vi "Append Goal.vi"(5 "Month":T1, 7 "YYYY":i32, 8 "error in (no error)":errorcluster, 9 "Goal Amount":dbl, 10 "Category_id":i32, 11 "Database in":refnum<class "Account History.lvclass">) -> (0 "error out":errorcluster, 2 "Added?":bool, 3 "Database out":refnum<class "Account History.lvclass">)   [LabVIEW 2018, in "Account History.lvclass"]
uses:
  Account History.lvclass
  Month.ctl
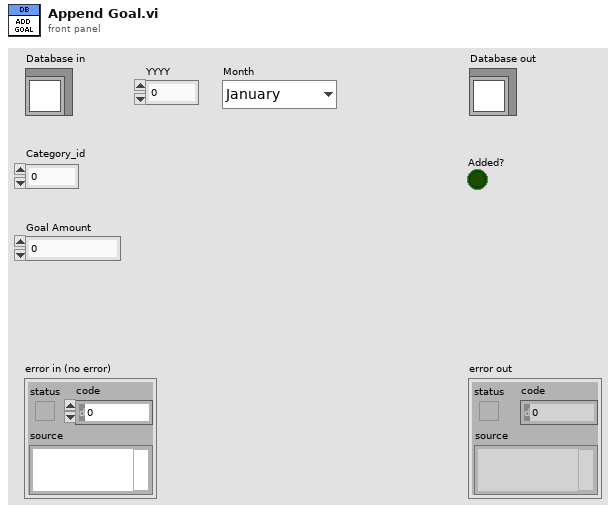
[diagram p1: front panel]
types:
  T1 = typedef "Account History.lvclass/Month.ctl" = enum16{"January", "February", "March", "April", "May", "June", "July", "August", "September", "October", "November", "December"}
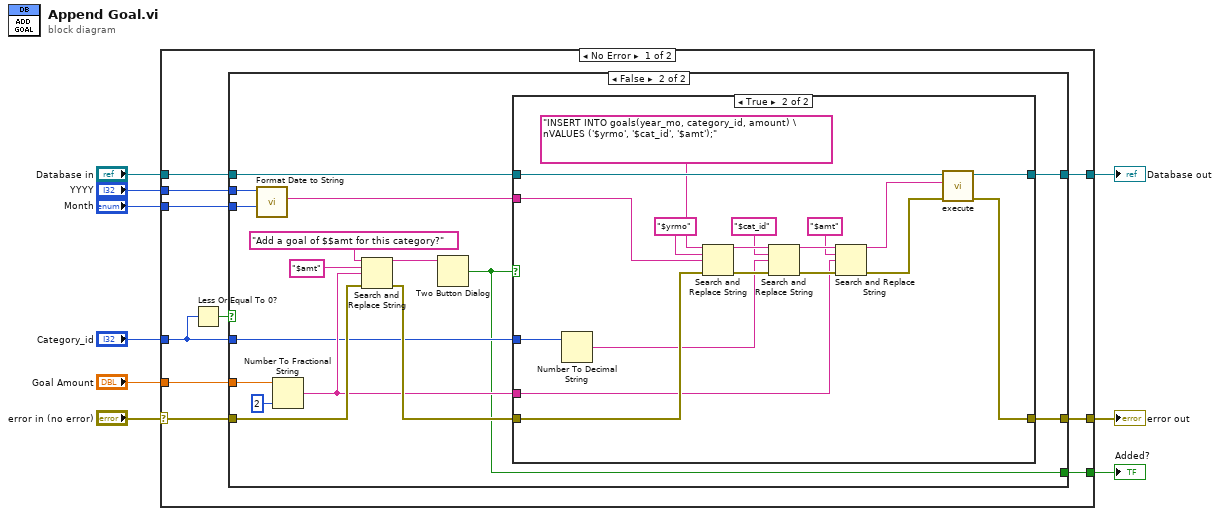
[diagram p0: block diagram]
diagram:
  n1 = case shown="No Error" "error in (no error)" {
    selector: "error in (no error)" -> [w15 w59]
    tunnel: [w17 w59] -> w8
    tunnel: [w18 w58] -> w6
    tunnel: "Database in" -> [w19 w58]
    tunnel: "Category_id" -> [w14 _]
    tunnel: "Goal Amount" -> [w16 _]
    tunnel: "YYYY" -> [w12 _]
    tunnel: "Month" -> [w11 _]
    tunnel: [w10 _] -> w1
    frame No Error {
      n2 = Less Or Equal To 0?(x=w14) -> (x <= 0?=w13:bool)
      n3 = case shown="False" w13 {
        tunnel: w19 -> [w21 w37]
        tunnel: [w21 w36] -> w18
        tunnel: [w20 w35] -> w17
        tunnel: w16 -> [_ w34]
        tunnel: w15 -> [w20 w32]
        tunnel: w14 -> [_ w26]
        tunnel: w12 -> [_ w25]
        tunnel: w11 -> [_ w24]
        tunnel: [_ w22] -> w10
        frame True {
        }
        frame False {
          n4 = call "Format Date to String.vi"("Month"=w24, "YYYY"=w25) -> ("Year-Mo"=w23:string)  [unwired: 9 in]
          n5 = Number To Fractional String(number=w34, precision (6)=i16 2) -> (F-format string=w27:string)  [unwired: 2 in]
          n6 = Search and Replace String(input string="Add a goal of $$amt for this category?", search string="$amt", replace string=w27, error in=w32) -> (result string=w30:string, error out=w31:errorcluster)  [unwired: 4 in, 2 out]
          n7 = Two Button Dialog(message=w30) -> (T button?=w22:bool)  [unwired: 2 in]
          n8 = case shown="True" w22 {
            tunnel: w37 -> [w39 w57]
            tunnel: [w39 w56] -> w36
            tunnel: [w38 w55] -> w35
            tunnel: w31 -> [w38 w52]
            tunnel: w26 -> [_ w44]
            tunnel: w27 -> [_ w41]
            tunnel: w23 -> [_ w40]
            frame False {
            }
            frame True {
              n9 = Number To Decimal String(number=w44) -> (decimal integer string=w43:string)  [unwired: 1 in]
              n10 = Search and Replace String(input string="INSERT INTO goals(year_mo, category_id, amount) \nVALUES ('$yrmo', '$cat_id', '$amt');", search string="$yrmo", replace string=w40, error in=w52) -> (result string=w51:string, error out=w50:errorcluster)  [unwired: 4 in, 2 out]
              n11 = Search and Replace String(input string=w51, search string="$cat_id", replace string=w43, error in=w50) -> (result string=w49:string, error out=w48:errorcluster)  [unwired: 4 in, 2 out]
              n12 = Search and Replace String(input string=w49, search string="$amt", replace string=w41, error in=w48) -> (result string=w42:string, error out=w47:errorcluster)  [unwired: 4 in, 2 out]
              n13 = call "execute.vi"("error in (no error)"=w47, "SQL query"=w42, "Database in"=w57) -> ("error out"=w55:errorcluster, "Database out"=w56:refnum<class "Account History.lvclass">)  [unwired: 7 in]
            }
          }
        }
      }
    }
    frame Error {
    }
  }
  "error out" <- w8
  "Database out" <- w6
  "Added?" <- w1
